vi "Sec_to_date_filename.vi"(0 "seconds":dbl) -> (1 "Year":string, 2 "Month":string, 3 "Day":string, 4 "Time":string)   [LabVIEW 2010]
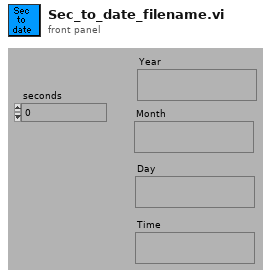
[diagram p1: front panel]
types:
  T1 = typedef "LVDateTimeRec.ctl" = cluster{"fractional second":dbl, "second":i32, "minute":i32, "hour":i32, "day of month":i32, "month":i32, "year":i32, "day of week":i32, "day of year":i32, "DST":i32}
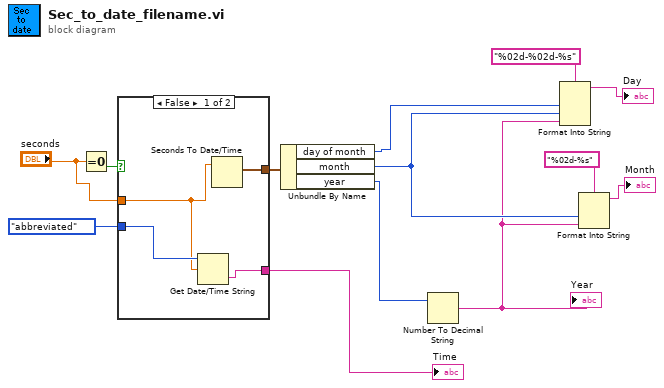
[diagram p0: block diagram]
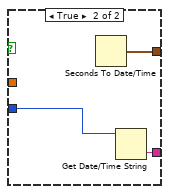
[diagram p2: hidden frame]
diagram:
  n1 = Equal To 0?(x="seconds") -> (x = 0?=w5:bool)
  n2 = case shown="False" w5 {
    tunnel: [w15 w18] -> w4
    tunnel: "seconds" -> [w14 _]
    tunnel: [w17 w20] -> w2
    tunnel: enum16{"short", "long", "abbreviated"}."abbreviated" ("date format (0)") -> [w16 w19]
    frame False {
      n3 = Get Date/Time String(date format (0)=w16, seconds (now)=w14) -> (time string=w17:string)  [unwired: 2 out]
      n4 = Seconds To Date/Time(time stamp (now)=w14) -> (date time rec=w15:T1)  [unwired: 1 out]
    }
    frame True {
      n5 = Seconds To Date/Time() -> (date time rec=w18:T1)  [unwired: 2 out]
      n6 = Get Date/Time String(date format (0)=w19) -> (time string=w20:string)  [unwired: 3 out]
    }
  }
  "Time" <- w2
  n7 = Unbundle By Name(w4) -> ("day of month"=w11:i32, "month"=w8:i32, "year"=w13:i32)
  n8 = Number To Decimal String(number=w13) -> (decimal integer string=w7:string)  [unwired: 1 out]
  "Year" <- w7
  n9 = Format Into String(format string="%02d-%02d-%s", w11, w8, w7) -> (resulting string=→"Day":string)  [unwired: 2 in, 1 out]
  n10 = Format Into String(format string="%02d-%s", w8, w7) -> (resulting string=→"Month":string)  [unwired: 2 in, 1 out]
